vi "2HP.vi"() -> (0 "DAQ Error":errorcluster)   [LabVIEW 2021]
doc: "Use this plug-in with the Nathan 7609 data acquisition system"
uses:
  Globals/Meas_global.vi
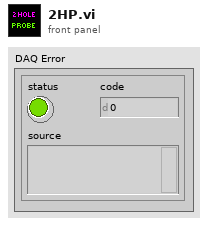
[diagram p1: front panel]
types:
  T1 = typedef "Analysis_info_cluster.ctl" = cluster{"Colour":u32, "Inst type":T2, "Inst name":string, "Symbol":string, "Code name":string, "Extra Info":string, "Inst Array":T3, "Extra Titles":string[], "Extra Values":string[], "U":dbl, "u^2":dbl, "u^3":dbl, "u^4":dbl, "Skew_u":dbl, "Kurt_u":dbl, "Sd Error in Mean":dbl, "% u'/U":dbl, "X":dbl, "Y":dbl, "Z":dbl, "Timescale integral Estimate":dbl, "Sd Error in Variance":dbl, "Calib File":path, "Calib Constants":dbl[], "Output Position":bool, "Stats":enum16{"None", "Basic", "Full"}, "Av Sampling Rate":dbl, "Av No of Samples":dbl, "Total Meas Time (s)":dbl, "ADAM Ch Name":string, "Max value":dbl, "Min value":dbl, "Req Sample Rate Hz":dbl, "Sync Delay Time (s)":dbl, "Ch No":i16, "Device":string, "Use Latest Calib":bool, "Port":string, "Metadata Ch Names":string[], "Metadata Ch Values":string[], "Label":string}
  T2 = typedef "Inst_type.ctl" = enum16{"Raw voltage", "Raw with zero offsetting", "Propeller anemometer", "Pressure Transducer", "Pitot-static tube", "Hot wire", "Cross wire 1", "Cross wire 2", "Generic Linear", "Generic Polynomial", "Generic BackPoly", "Fast FID", "Thermocouple", "Cold wire", "Pulsed Wire", "LDA Vel", "LDA Tran time", "LDA Arr time", "Microphone"}
  T3 = typedef "Instrument_Array.ctl" = enum16{"PWA", "LDA", "Analogue"}
  T4 = typedef "Setup.ctl" = enum16{"Run Program", "Show Setup", "Save Current Setup", "Setup Front Panel"}
  T5 = typedef "Device ID port info.ctl" = cluster{"Ch No":i16[], "Req Sampling Rate":dbl[], "Port":string, "Index":i32[]}
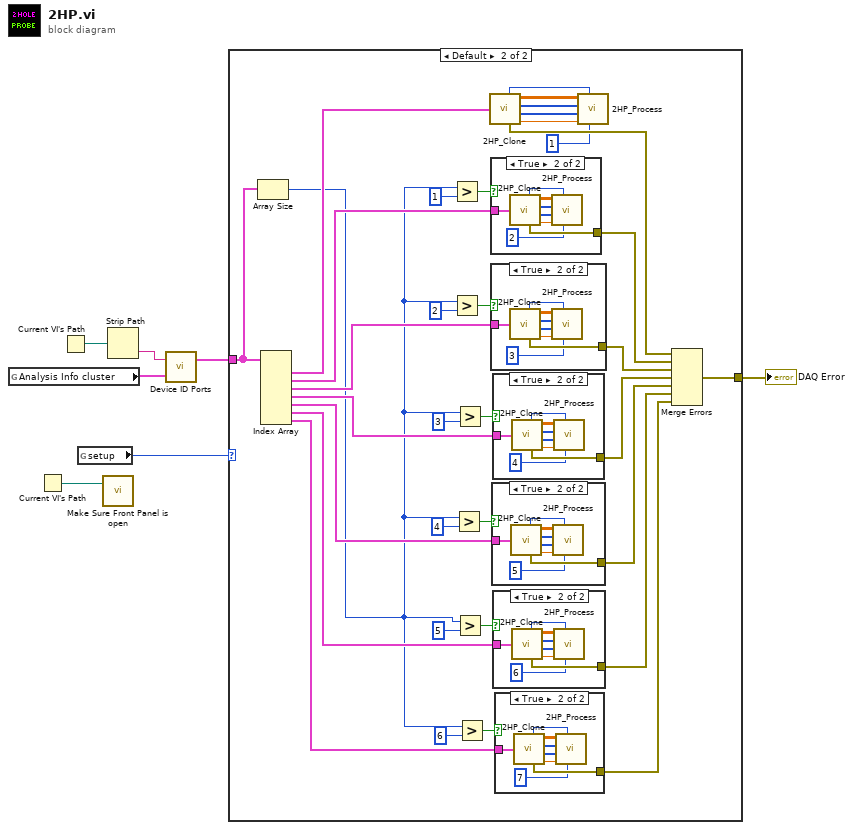
[diagram p0: block diagram]
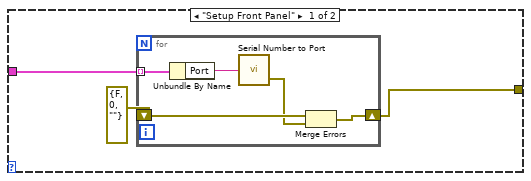
[diagram p2: hidden frame]
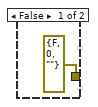
[diagram p3: hidden frame]
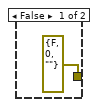
[diagram p4: hidden frame]
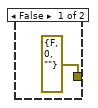
[diagram p5: hidden frame]
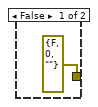
[diagram p6: hidden frame]
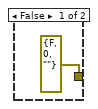
[diagram p7: hidden frame]
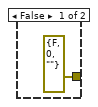
[diagram p8: hidden frame]
diagram:
  n1 = global read "Meas_global.vi" "Analysis Info cluster"() -> (w3:T1[])
  n2 = Current VI's Path() -> (path=w5:path)
  n3 = Current VI's Path() -> (path=w2:path)
  n4 = global read "Meas_global.vi" "setup"() -> (w6:T4)
  n5 = call "Make Sure Front Panel is open.vi"("path"=w5) -> ()
  n6 = Strip Path(path=w2) -> (name=w4:string)  [unwired: 1 out]
  n7 = call "Device ID Ports.vi"("Analysis Info cluster"=w3, "Device ID"=w4) -> ("Device port info"=w1:T5[])  [unwired: 1 out]
  n8 = case shown="Default" w6 {
    tunnel: w1 -> [w10 w17]
    tunnel: [w8 w20] -> w7
    frame "Setup Front Panel" {
      n9 = for {
        tunnel: w10 -> [w15] mode=indexing
        shift-right: [w11] -> w8
        shift-left: errorcluster {"status"=FALSE, "code"=0, "source"=""} ("error IO") -> [w13]
        n10 = Unbundle By Name(w15) -> ("Port"=w14:string)
        n11 = call "Serial Number to Port.vi"("Port In"=w14) -> ("error out"=w12:errorcluster)  [unwired: 1 out]
        n12 = Merge Errors(w13, w12) -> (w11:errorcluster)
      }
    }
    frame Default {
      n13 = Array Size(array=w17) -> (size(s)=w16:i32)
      n14 = Index Array(array=w17) -> (element #1=w46:T5, element #2=w33:T5, element #3=w32:T5, element #4=w31:T5, element #5=w30:T5, element #6=w29:T5, element #7=w28:T5)  [unwired: 7 in]
      n15 = Greater?(x=w16, y=1) -> (0:w44:bool)
      n16 = Greater?(x=w16, y=2) -> (0:w43:bool)
      n17 = Greater?(x=w16, y=4) -> (0:w39:bool)
      n18 = Greater?(x=w16, y=3) -> (0:w40:bool)
      n19 = Greater?(x=w16, y=5) -> (0:w36:bool)
      n20 = Greater?(x=w16, y=6) -> (0:w35:bool)
      n21 = call "2HP_Clone.vi"("Single 2HP"=w46) -> ("Serial number"=w19:u32, "DAQ Error"=w26:errorcluster, "All samples out"=w47:sgl[][], "Ch No"=w48:i16[], "Index"=w49:i32[], "Sampling Rate Hz"=w50:dbl)
      n22 = case shown="True" w44 {
        tunnel: w33 -> [_ w100]
        tunnel: [errorcluster {"status"=FALSE, "code"=0, "source"=""} ("DAQ Error") w99] -> w27
        frame False {
        }
        frame True {
          n23 = call "2HP_Clone.vi"("Single 2HP"=w100) -> ("Serial number"=w97:u32, "DAQ Error"=w99:errorcluster, "All samples out"=w104:sgl[][], "Ch No"=w103:i16[], "Index"=w102:i32[], "Sampling Rate Hz"=w101:dbl)
          n24 = call "2HP_Process.vi"("All samples in"=w104, "Serial number"=w97, "2HP Ch No"=w103, "Analysis info Index"=w102, "Probe Number"=2, "Sampling Rate"=w101) -> ()  [unwired: 3 in]
        }
      }
      n25 = case shown="True" w43 {
        tunnel: w32 -> [_ w91]
        tunnel: [errorcluster {"status"=FALSE, "code"=0, "source"=""} ("DAQ Error") w90] -> w25
        frame False {
        }
        frame True {
          n26 = call "2HP_Clone.vi"("Single 2HP"=w91) -> ("Serial number"=w88:u32, "DAQ Error"=w90:errorcluster, "All samples out"=w95:sgl[][], "Ch No"=w94:i16[], "Index"=w93:i32[], "Sampling Rate Hz"=w92:dbl)
          n27 = call "2HP_Process.vi"("All samples in"=w95, "Serial number"=w88, "2HP Ch No"=w94, "Analysis info Index"=w93, "Probe Number"=3, "Sampling Rate"=w92) -> ()  [unwired: 3 in]
        }
      }
      n28 = case shown="True" w39 {
        tunnel: w30 -> [_ w73]
        tunnel: [errorcluster {"status"=FALSE, "code"=0, "source"=""} ("DAQ Error") w72] -> w23
        frame False {
        }
        frame True {
          n29 = call "2HP_Clone.vi"("Single 2HP"=w73) -> ("Serial number"=w70:u32, "DAQ Error"=w72:errorcluster, "All samples out"=w77:sgl[][], "Ch No"=w76:i16[], "Index"=w75:i32[], "Sampling Rate Hz"=w74:dbl)
          n30 = call "2HP_Process.vi"("All samples in"=w77, "Serial number"=w70, "2HP Ch No"=w76, "Analysis info Index"=w75, "Probe Number"=5, "Sampling Rate"=w74) -> ()  [unwired: 3 in]
        }
      }
      n31 = case shown="True" w40 {
        tunnel: w31 -> [_ w82]
        tunnel: [errorcluster {"status"=FALSE, "code"=0, "source"=""} ("DAQ Error") w81] -> w24
        frame False {
        }
        frame True {
          n32 = call "2HP_Clone.vi"("Single 2HP"=w82) -> ("Serial number"=w79:u32, "DAQ Error"=w81:errorcluster, "All samples out"=w86:sgl[][], "Ch No"=w85:i16[], "Index"=w84:i32[], "Sampling Rate Hz"=w83:dbl)
          n33 = call "2HP_Process.vi"("All samples in"=w86, "Serial number"=w79, "2HP Ch No"=w85, "Analysis info Index"=w84, "Probe Number"=4, "Sampling Rate"=w83) -> ()  [unwired: 3 in]
        }
      }
      n34 = case shown="True" w36 {
        tunnel: w29 -> [_ w64]
        tunnel: [errorcluster {"status"=FALSE, "code"=0, "source"=""} ("DAQ Error") w63] -> w22
        frame False {
        }
        frame True {
          n35 = call "2HP_Clone.vi"("Single 2HP"=w64) -> ("Serial number"=w61:u32, "DAQ Error"=w63:errorcluster, "All samples out"=w68:sgl[][], "Ch No"=w67:i16[], "Index"=w66:i32[], "Sampling Rate Hz"=w65:dbl)
          n36 = call "2HP_Process.vi"("All samples in"=w68, "Serial number"=w61, "2HP Ch No"=w67, "Analysis info Index"=w66, "Probe Number"=6, "Sampling Rate"=w65) -> ()  [unwired: 3 in]
        }
      }
      n37 = case shown="True" w35 {
        tunnel: w28 -> [_ w55]
        tunnel: [errorcluster {"status"=FALSE, "code"=0, "source"=""} ("DAQ Error") w54] -> w21
        frame False {
        }
        frame True {
          n38 = call "2HP_Clone.vi"("Single 2HP"=w55) -> ("Serial number"=w52:u32, "DAQ Error"=w54:errorcluster, "All samples out"=w59:sgl[][], "Ch No"=w58:i16[], "Index"=w57:i32[], "Sampling Rate Hz"=w56:dbl)
          n39 = call "2HP_Process.vi"("All samples in"=w59, "Serial number"=w52, "2HP Ch No"=w58, "Analysis info Index"=w57, "Probe Number"=7, "Sampling Rate"=w56) -> ()  [unwired: 3 in]
        }
      }
      n40 = call "2HP_Process.vi"("All samples in"=w47, "Serial number"=w19, "2HP Ch No"=w48, "Analysis info Index"=w49, "Probe Number"=1, "Sampling Rate"=w50) -> ()  [unwired: 3 in]
      n41 = Merge Errors(w26, w27, w25, w24, w23, w22, w21) -> (w20:errorcluster)
    }
  }
  "DAQ Error" <- w7
